vi "Get Channels and Refresh Tree.vi"(7 "Item Ref in":T9 format="%.0x", 8 "error in (no error)":errorcluster, 10 "data":T1, 11 "TreeControl in":refnum<vi>) -> (0 "error out":errorcluster, 1 "Enum Strings":cluster{"name":string, string}[](array[cluster]), 2 "Enums":T2[](array[typedef]), 3 "SLSC Output Tree":T8(array[cluster]), 4 "SLSC EDS module out":T1, 5 "Item Ref out":T9 format="%.0x")   [LabVIEW 2020]
uses:
  SLSC UI API/SLSC Tree Control.lvlib
  SLSC CD API/SLSC CD System Explorer/SLSC CD System Explorer.lvlib
  SLSC EDS System Explorer.lvlib
  Shared/Constants.vi
  Shared/SLSC EDS Shared.lvlib
  <vilib>/NI VeriStand/Custom Device API/Custom Device Item Ref.ctl
  <vilib>/NI VeriStand/Custom Device API/Custom Device API.lvlib
  SLSC EDS API/JSON parsing/enum.ctl
  SLSC EDS API/JSON parsing/command.ctl
  SLSC EDS API/JSON parsing/property.ctl
  SLSC EDS API/JSON parsing/physicalChannel.ctl
  SLSC EDS API/JSON parsing/scale.ctl
  SLSC EDS API/JSON parsing/register.ctl
  SLSC EDS API/JSON parsing/EDSjsonStructure.ctl
panel:
  # "not working\nregisterMap->registers->initialValue"
  # "not working\nregisterMap->registers->initialValue"
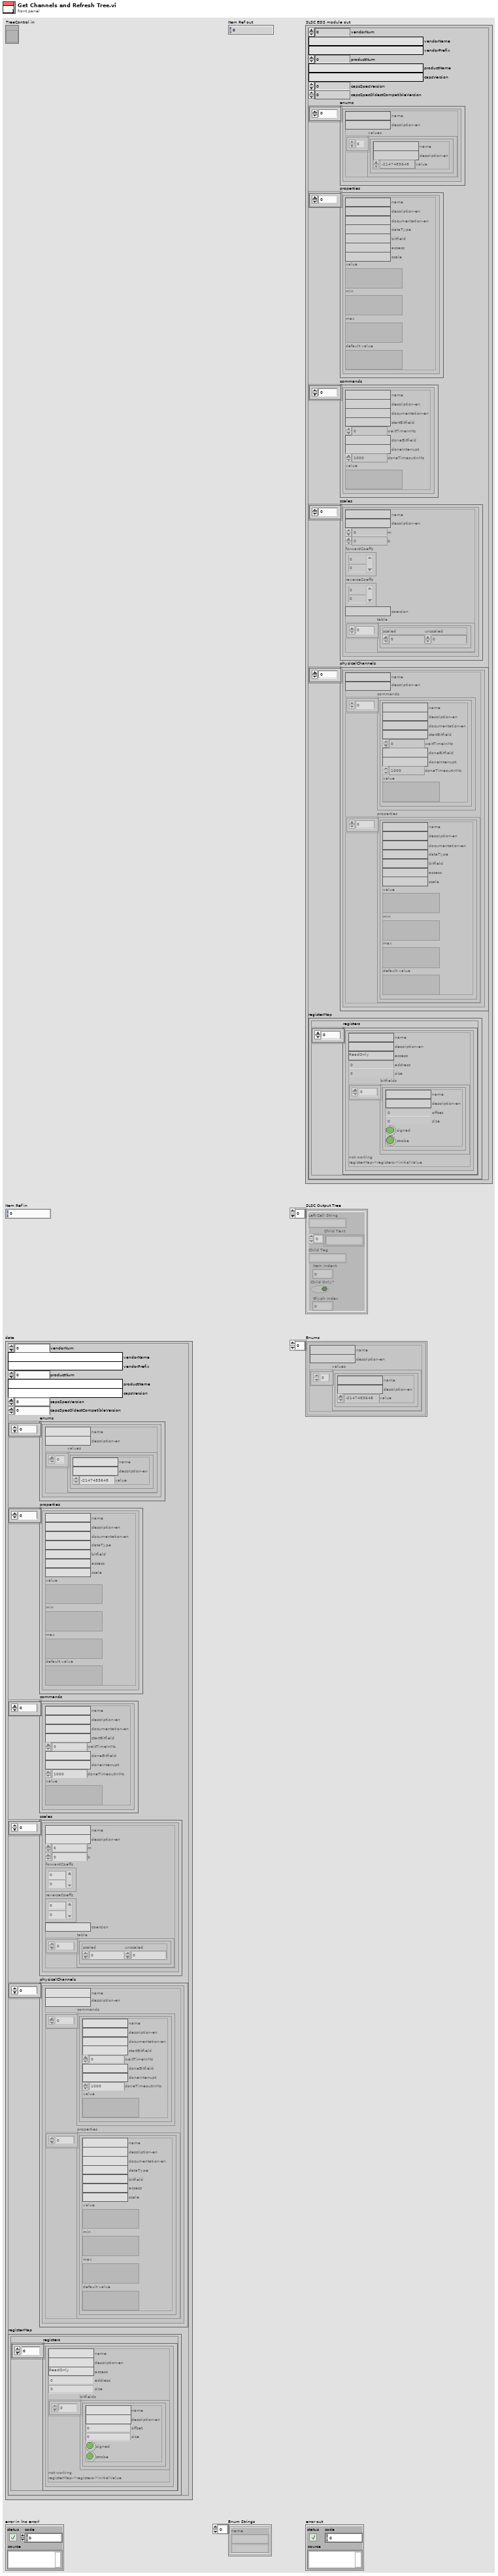
[diagram p1: front panel]
types:
  T1 = typedef "EDSjsonStructure.ctl" = cluster{"vendorNum":u32, "vendorName":string, "vendorPrefix":string, "productNum":u32, "productName":string, "capsVersion":string, "capsSpecVersion":u32, "capsSpecOldestCompatibleVersion":u32, "enums":T2[], "properties":T3[], "commands":T4[], "scales":T5[], "physicalChannels":T6[], "registerMap":cluster{"registers":T7[]}}
  T2 = typedef "enum.ctl" = cluster{"name":string, "description-en":string, "values":cluster{"name":string, "description-en":string, "value":i32}[]}
  T3 = typedef "property.ctl" = cluster{"name":string, "description-en":string, "documentation-en":string, "dataType":string, "bitfield":string, "access":string, "scale":string, "value":variant, "min":variant, "max":variant, "default value":variant}
  T4 = typedef "command.ctl" = cluster{"name":string, "description-en":string, "documentation-en":string, "startBitfield":string, "waitTimeInMs":i32, "doneBitfield":string, "doneInterrupt":string, "doneTimeoutInMs":i32, "value":variant}
  T5 = typedef "scale.ctl" = cluster{"name":string, "description-en":string, "m":dbl, "b":dbl, "forwardCoeffs":dbl[], "reverseCoeffs":dbl[], "coercion":string, "table":cluster{"scaled":dbl, "unscaled":dbl}[]}
  T6 = typedef "physicalChannel.ctl" = cluster{"name":string, "description-en":string, "commands":T4[], "properties":T3[]}
  T7 = typedef "register.ctl" = cluster{"name":string, "description-en":string, "access":string, "address":u32, "size":u32, "bitfields":cluster{"name":string, "description-en":string, "offset":u32, "size":u32, "signed":bool, "strobe":bool}[]}
  T8 = cluster{"Left Cell String":string, "Child Text":string[], "Child Tag":string, "Item Indent":i32, "Child Only?":bool, "Glyph Index":i32}[]
  T9 = typedef "Custom Device API.lvlib/Custom Device Item Ref.ctl" = u64
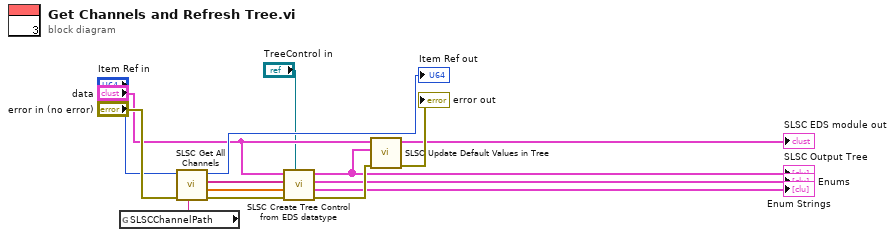
[diagram p0: block diagram]
diagram:
  n1 = global read "Constants.vi" "SLSCChannelPath"() -> (w11:string)
  n2 = call "SLSC Get All Channels.vi"("SLSCChannelPath"=w11, "error in (no error)"="error in (no error)", "Item Ref in"="Item Ref in") -> ("error out"=w7:errorcluster, "Channel Values"=w9:dbl[], "TreeItem Channels"=w8:string[], "Item Ref out"=→"Item Ref out":T9)  [unwired: 5 in]
  n3 = call "SLSC Create Tree Control from EDS datatype.vi"("Property Tree"="TreeControl in", "error in (no error)"=w7, "Channel Values"=w9, "Properties to enable"=w8, "SLSC EDS module"="data") -> ("error out"=w13:errorcluster, "Enum Strings"=→"Enum Strings":cluster{"name":string, string}[], "Enums"=→"Enums":T2[], "SLSC Output Tree"=w2:T8)  [unwired: 3 in]
  "SLSC Output Tree" <- w2
  n4 = call "SLSC Update Default Values in Tree.vi"("error in (no error)"=w13, "SLSC Output Tree"=w2, "SLSC EDS module in"="data") -> ("error out"=→"error out":errorcluster, "SLSC EDS module out"=→"SLSC EDS module out":T1)  [unwired: 7 in]
